vi "PGPASS.Read.vi"(8 "error in":errorcluster) -> (0 "error out":errorcluster, 3 "Connections":T1[](array[typedef]))   [LabVIEW 2019, in "PGPASS.lvlib"]
uses:
  PGPASS.lvlib
  PGPASS.Connection Information.ctl
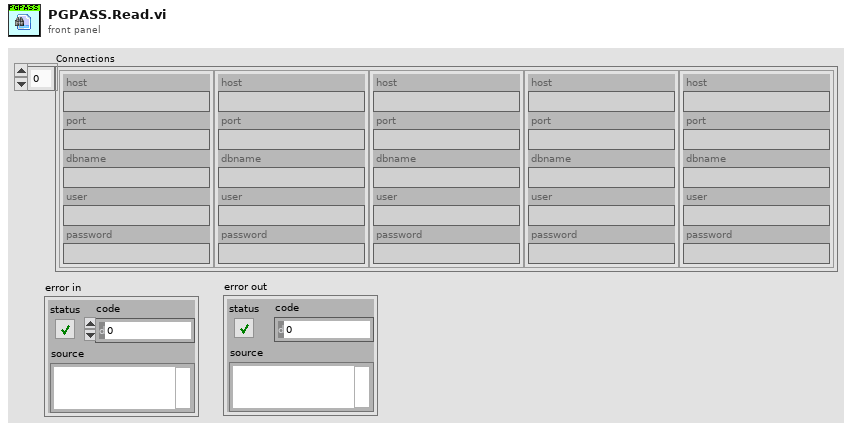
[diagram p1: front panel]
types:
  T1 = typedef "PGPASS.lvlib/PGPASS.Connection Information.ctl" = cluster{"host":string, "port":string, "dbname":string, "user":string, "password":string}
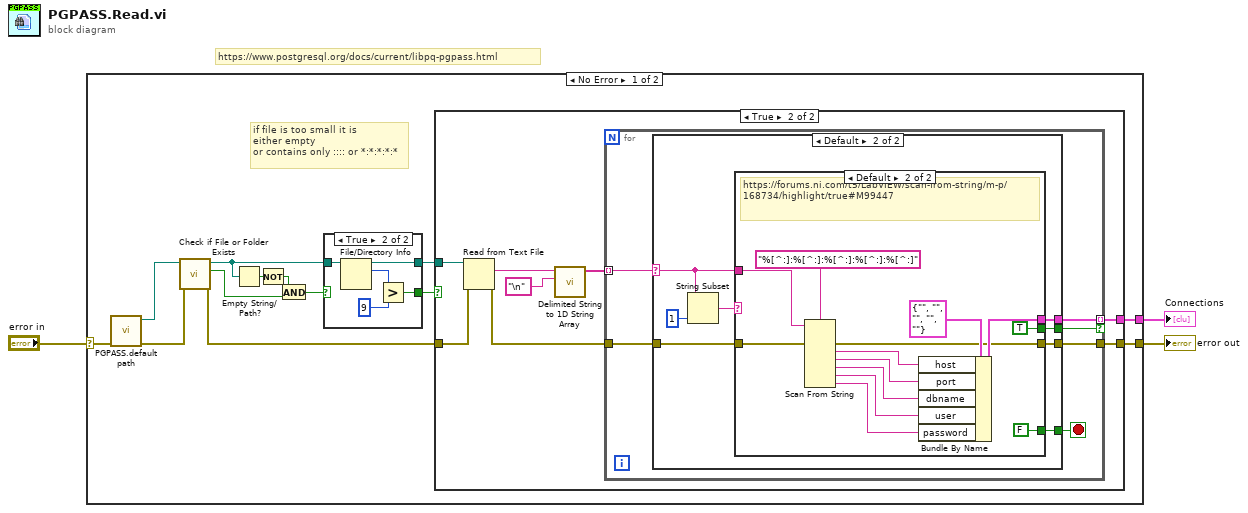
[diagram p0: block diagram]
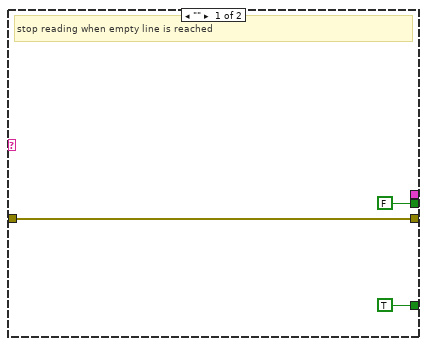
[diagram p3: hidden frame]
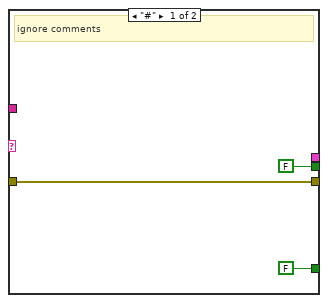
[diagram p4: hidden frame]
diagram:
  # "https://www.postgresql.org/docs/current/libpq-pgpass.html"
  n1 = case shown="No Error" "error in" {
    selector: "error in" -> [w14 w66]
    tunnel: [w16 w66] -> w1
    tunnel: [w15 _] -> w2
    frame No Error {
      # "if file is too small it is\neither empty\nor contains only :::: or *:*:*:*:*"
      n2 = call "PGPASS.default path.vi"("error in (no error)"=w14) -> ("error out"=w7:errorcluster, "PGPASS path"=w11:path)  [unwired: 9 in]
      n3 = call <vilib>:"Check if File or Folder Exists.vi"("error in (no error)"=w7, "path"=w11) -> ("error out"=w6:errorcluster, "file or folder exists?"=w8:bool, "dup path"=w10:path)  [unwired: 7 in]
      n4 = Empty String/Path?(string/path=w10) -> (empty?=w9:bool)
      n5 = Not(x=w9) -> (.not. x?=w5:bool)
      n6 = And(x=w5, y=w8) -> (x .and. y?=w4:bool)
      n7 = case shown="True" w4 {
        selector: w4 -> [w59 _]
        tunnel: w10 -> [w60 w65]
        tunnel: [w60 w64] -> w12
        tunnel: [w59 w61] -> w13
        frame False {
        }
        frame True {
          n8 = File/Directory Info(path=w65) -> (path out=w64:path, size=w63:i64)  [unwired: 1 in, 5 out]
          n9 = Greater?(x=w63, y=i64 9) -> (0:w61:bool)
        }
      }
      n10 = case shown="True" w13 {
        tunnel: [w17 w22] -> w16
        tunnel: w6 -> [w17 w25]
        tunnel: [_ w23] -> w15
        tunnel: w12 -> [_ w24]
        frame False {
        }
        frame True {
          n11 = Read from Text File(file (use dialog)=w24, error in=w25) -> (text=w19:string, error out=w20:errorcluster)  [unwired: 2 in, 2 out]
          n12 = call <vilib>:"Delimited String to 1D String Array.vi"("delimiter"="\n" ("delimiter (Tab)"), "delimited string"=w19) -> ("string array"=w21:string[])  [unwired: 9 in]
          n13 = for {
            tunnel: [w31] -> w23 mode=indexing if=w26
            tunnel: w20 -> [w30]
            tunnel: [w29] -> w22
            tunnel: w21 -> [w28] mode=indexing
            stop <- w27 stop-if-true
            n14 = case shown="Default" w28 {
              selector: w28 -> [_ w39]
              tunnel: [_ w42] -> w31
              tunnel: w30 -> [w34 w41]
              tunnel: [w34 w40] -> w29
              tunnel: [TRUE w36] -> w27
              tunnel: [FALSE w35] -> w26
              frame "" {
                # "stop reading when empty line is reached"
              }
              frame Default {
                n15 = String Subset(string=w39, length (rest)=1 ("length (rest)")) -> (substring=w37:string)  [unwired: 1 in]
                n16 = case shown="Default" w37 {
                  tunnel: [_ w58] -> w42
                  tunnel: w41 -> [w45 w52]
                  tunnel: [w45 w51] -> w40
                  tunnel: w39 -> [_ w49]
                  tunnel: [FALSE FALSE] -> w36
                  tunnel: [FALSE TRUE] -> w35
                  frame "#" {
                    # "ignore comments"
                  }
                  frame Default {
                    # "https://forums.ni.com/t5/LabVIEW/scan-from-string/m-p/168734/highlight/true#M99447"
                    n17 = Scan From String(format string="%[^:]:%[^:]:%[^:]:%[^:]:%[^:]", input string=w49, error in=w52) -> (error out=w51:errorcluster, output 1=w55:string, output 2=w54:string, output 3=w53:string, output 4=w50:string, output 5=w46:string)  [unwired: 6 in, 2 out]
                    n18 = Bundle By Name(cluster=T1 {"host"="", "port"="", "dbname"="", "user"="", "password"=""} ("Connection Information"), "host"=w55, "port"=w54, "dbname"=w53, "user"=w50, "password"=w46) -> (w58:T1)
                  }
                }
              }
            }
          }
        }
      }
    }
    frame Error {
    }
  }
  "error out" <- w1
  "Connections" <- w2
